vi "Dashboard Main.vi"() -> ()   [LabVIEW 2019]
uses:
  Program Files (x86)/National Instruments/LabVIEW 2019/examples/Design Patterns/Queued Message Handler/support/QMH Fundamentals - Message Cluster.ctl
  <vilib>/Utility/miscctls.llb/LVRowAndColumnTypeDef.ctl
  <vilib>/event_ctls.llb/eventvkey.ctl
  src robot/TypeDefs/Falcon Temperatures.ctl
  <vilib>/Rock Robotics/WPI/Dashboard/WPI_DashboardLogging Global.vi
  <vilib>/Rock Robotics/Network Tables/NT Read Numeric Array.vi
  <vilib>/Rock Robotics/Network Tables/NT Read Boolean.vi
  <vilib>/Rock Robotics/Network Tables/NT Write Boolean.vi
  Personalities Tool/Personalities Tool.lvlib
  91361502-ee7e-4c80-8d6f-41942abc4405.vi
panel:
  in  "Mini View Toolbar":bool
  in  "Mini View Button":bool
  out "Boolean 5":bool
  in  "Boolean 4":bool
  in  "Developer Settings":bool
  in  "Match Ready":bool
  in  "Left Sidebar Expanded":bool
  in  "Left Sidebar Mini":bool
  in  "Minimized Toolbar Button":bool
  out "Tab Control 2":enum32{"Page 1", "Page 2"}(tab)
  out "Numeric 3":dbl
  out "String 5":string
  out "New Throttle 2":bool
  out "Highest Temp Label 3":string
  out "Highest Temp Label 4":string
  in  "Flywheel Velocity - 2":bool
  in  "Flywheel Velocity Plus 2":bool
  out "String 7":string
  out "String 8":string
  out "String 6":string
  out "Numeric 2":dbl
  out "String":string
  out "Widger Manager":enum32{"Page 1", "Page 2"}(tab)
  out "String 2":string
  out "String 3":string
  in  "Flywheel Velocity Plus":bool
  in  "Flywheel Velocity -":bool
  out "Highest Temp Label":string
  out "String 4":string
  out "Highest Temp Label 2":string
  out "New Throttle":bool
  in  "Boolean":bool
  out "Tab Control":enum32{"Page 1", "Page 3", "Page 2"}(tab)
  in  "Exanded View Toolbar":bool
  in  "stop 2":bool
  out "# elements in queue 2":i32
  out "Elapsed Time (s)":dbl
  out "# elements in queue":i32
  in  "TCP":refnum<k5>
  in  "Rec Mode":enum32{"Stop", "Record", "Playback"}(radio)
  out "Robot IP":string
  out "Image Message":string="Timeout in Camera Communications"
  in  "Dashboard Tab":T1(tab)
  out "Right follow":dbl
  out "Left follow":dbl
  out "Turret":dbl
  out "Right Lead":dbl
  out "Left lead":dbl
  out "Flywheel":dbl
  out "Flywheel Velocity":dbl
  in  "Select Auto":string(combo)="Select Autonomous ..."
  out "NT Connection":bool
  out "Mode":T2(ring)=enum."Auto Disabled"
  out "Accelerator":dbl format="%#_6f"
  in  "Shooter Trim +":bool
  in  "DB/String 9":string
  in  "DB/String 8":string
  in  "DB/String 7":string
  in  "DB/String 6":string
  in  "DB/String 5":string
  in  "DB/String 4":string
  in  "DB/String 3":string
  in  "DB/String 2":string
  in  "DB/String 1":string
  in  "DB/String 0":string
  in  "DB/Slider 0":dbl(slide) scale=0.0..5.0
  in  "DB/Slider 1":dbl(slide) scale=0.0..5.0
  in  "DB/Slider 2":dbl(slide) scale=0.0..5.0
  in  "DB/Slider 3":dbl(slide) scale=0.0..5.0
  out "DB/LED 3":bool
  out "DB/LED 2":bool
  out "DB/LED 1":bool
  out "DB/LED 0":bool
  in  "DB/Button 3":bool
  in  "DB/Button 2":bool
  in  "DB/Button 1":bool
  in  "DB/Button 0":bool caption="New Name"
  in  "Launch Personalities Tool":bool
  in  "Test Slider":dbl(slide) scale=0.0..100.0 scale format="%#_3g"
  in  "On/Off":bool caption="Solenoid"
  in  "Test Name":u16(ring) items=["Select the test to run..."]
  in  "Test Tree":string(tree)
  in  "Motor":cluster{"Value":dbl, "Enable":bool} {"Value" scale=-1.0..1.0 scale format="%#_3g"}
  out "Progress":T3 {"Test Progress" scale=0.0..100.0}
  in  "Rev/Fwd":cluster{"Forward":bool, "Reverse":bool}
  in  "Test Ring":u16(ring) items=["Monochrome", "Color"]
  out "Cmd Status":string
  in  "Execute Command":bool
  in  "Command Params":string[][](table)
  in  "Command Selection":i32(listbox)
  in  "CheckList":i32(listbox)
  out "Tree":string(tree)
  # "o"
  # "F"
  # "o"
  # "F"
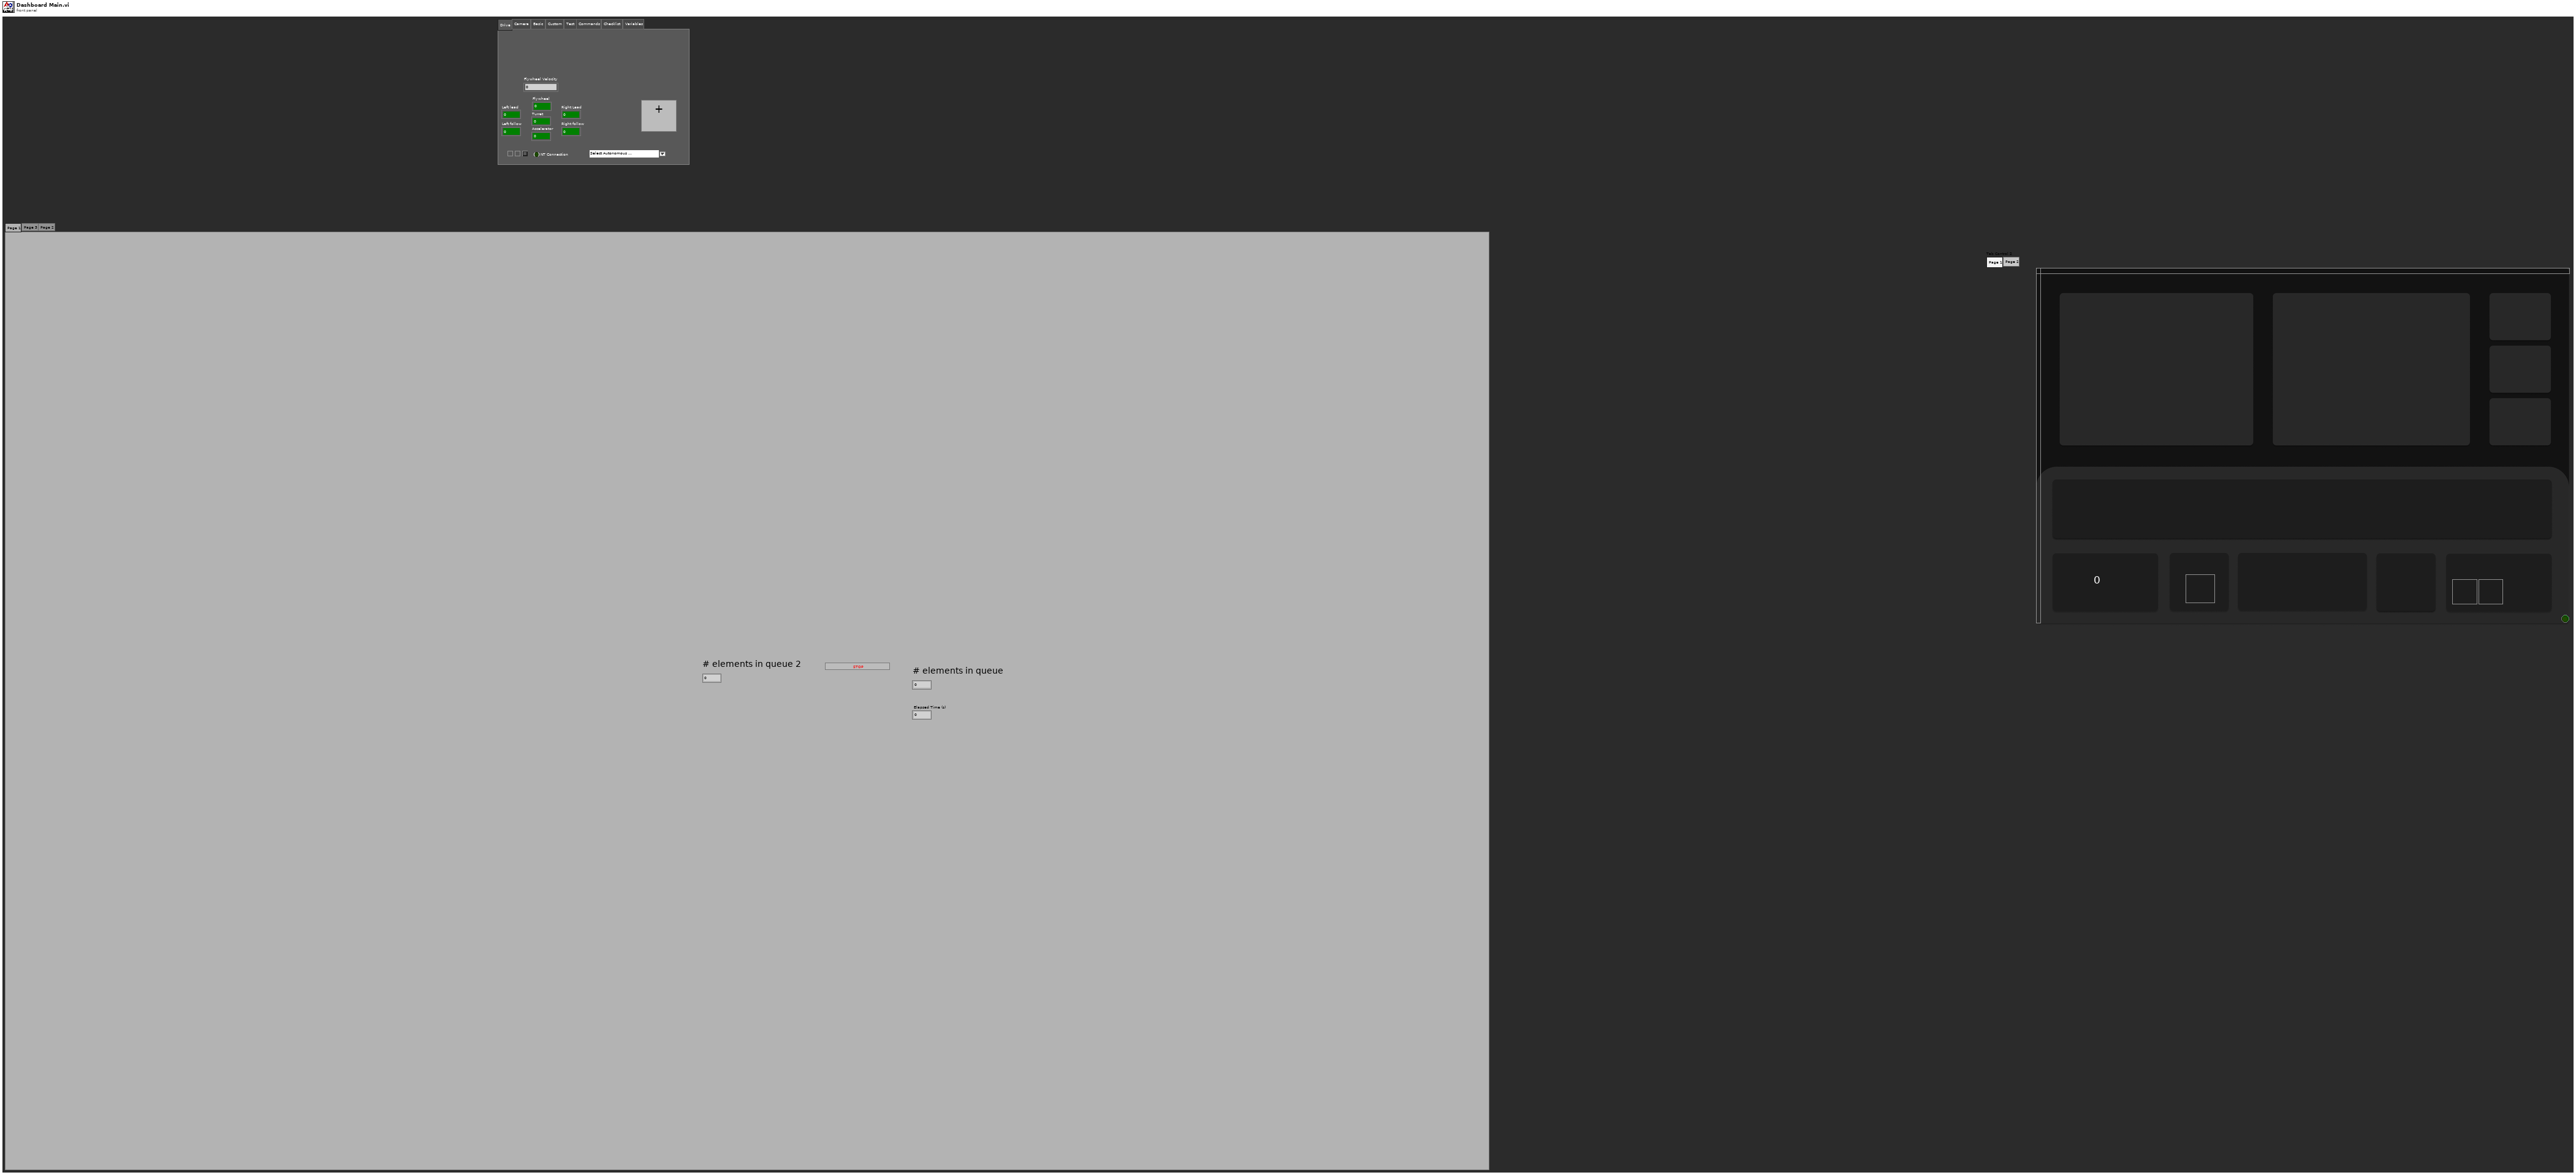
[diagram p1: front panel]
types:
  T1 = enum32{"Drive", "Camera", "Basic", "Custom", "Test", "Commands", "Checklist", "Variables"}
  T2 = enum8{"Tele-Op Disabled", "Tele-Op Enabled", "Auto Disabled", "Auto Enabled", "Test Disabled", "Test Enabled", "Disconnected", "No Code", "E-Stop"}
  T3 = cluster{"Test Progress":u8, "Test Progress Text":string}
  T4 = typedef "QMH Fundamentals - Message Cluster.ctl" = cluster{"Message":string, "Message Data":variant}
  T5 = cluster{"IDs":cluster{"RPC field ID":u16, "Unique ID":u16}, "String":string}
  T6 = typedef "Falcon Temperatures.ctl" = enum16{"Accelerator", "Turret", "Flywheel", "Right follow", "Right lead", "Left follow", "Left lead"}
  T7 = cluster{"Error Strings":string, "Disable Counts":cluster{u16, u16}, "Rail Faults":cluster{u16, u16, u16}, "Robot IP":string, "DB Mode":u8, "Event Info":cluster{"Name":string, "Type":u8, "Number":u16, "Replay":u8}}
  T8 = cluster{"Storage":cluster{"Disk Free":u64, "RAM Block":u32, "RAM free":u32}, "CPU Utilization":cluster{"CPU % ISR":sgl, "CPU % Time Crit":sgl, "CPU % Timed Str":sgl, "CPU % High":sgl, "CPU % Above":sgl, "CPU % Normal":sgl, "CPU % Low":sgl}, "CAN":cluster{"% Bus Utilization":sgl, "Bus Off Cnt":u32, "TX_FIFO Full Cnt":u32, "Receive Error Cnt":u8, "Transmit Error Cnt":u8}, "HID":cluster{"HID Outputs":u32, "Rumble Low":u16, "Rumble High":u16}[]}
  T9 = cluster{"Status bits":cluster{"Test Mode":bool, "Autonomous":bool, "Enabled":bool, "Code Start":bool, "Brownout":bool, "Reserved 2":bool, "Reserved 3":bool, "E-Stop":bool}, "Code Trace":cluster{"Disabled":bool, "TeleOp":bool, "Auto":bool, "Test":bool}, "Controller Type":enum16{"unknown", "cRIO", "roboRio"}, "Code?":enum16{"unknown", "noCode", "code"}, "Battery V":dbl}
  T10 = cluster{"Operation":enum16{"Update", "Clear"}, "Color Box":u32}[]
  T11 = typedef "eventvkey.ctl" = enum16{"ASCII", "Enter", "Return", "Shift", "Ctrl", "Alt", "Cmd", "Opt", "Caps", "NumLock", "Clear", "Break", "Up", "Down", "Left", "Right", "Insert", "Delete", "Home", "End", "PageUp", "PageDown", "Escape", "Help", "Pause", "ScrollLock", "F1", "F2", "F3", "F4", "F5", "F6", "F7", "F8", "F9", "F10", "F11", "F12", "F13", "F14", "F15", "F16", "F17", "F18", "F19", "F20", "F21", "F22", "F23", "F24", "Play", "VolumeUp", "VolumeDown", "Mute", "Two Byte Char"}
  T12 = cluster{"Image Size":bool, "Image Type":bool, "Pixel Value":bool, "ROI Information":bool, "Zoom Factor":bool}
  T13 = cluster{"Operation":enum16{"Update", "Clear"}, "Color Box":u32}
  T14 = typedef "LVRowAndColumnTypeDef.ctl" = cluster{"Row":i32, "Column":i32}
  T15 = cluster{"Shift":bool, "Ctrl":bool, "Alt":bool, "Cmd":bool, "Opt":bool}
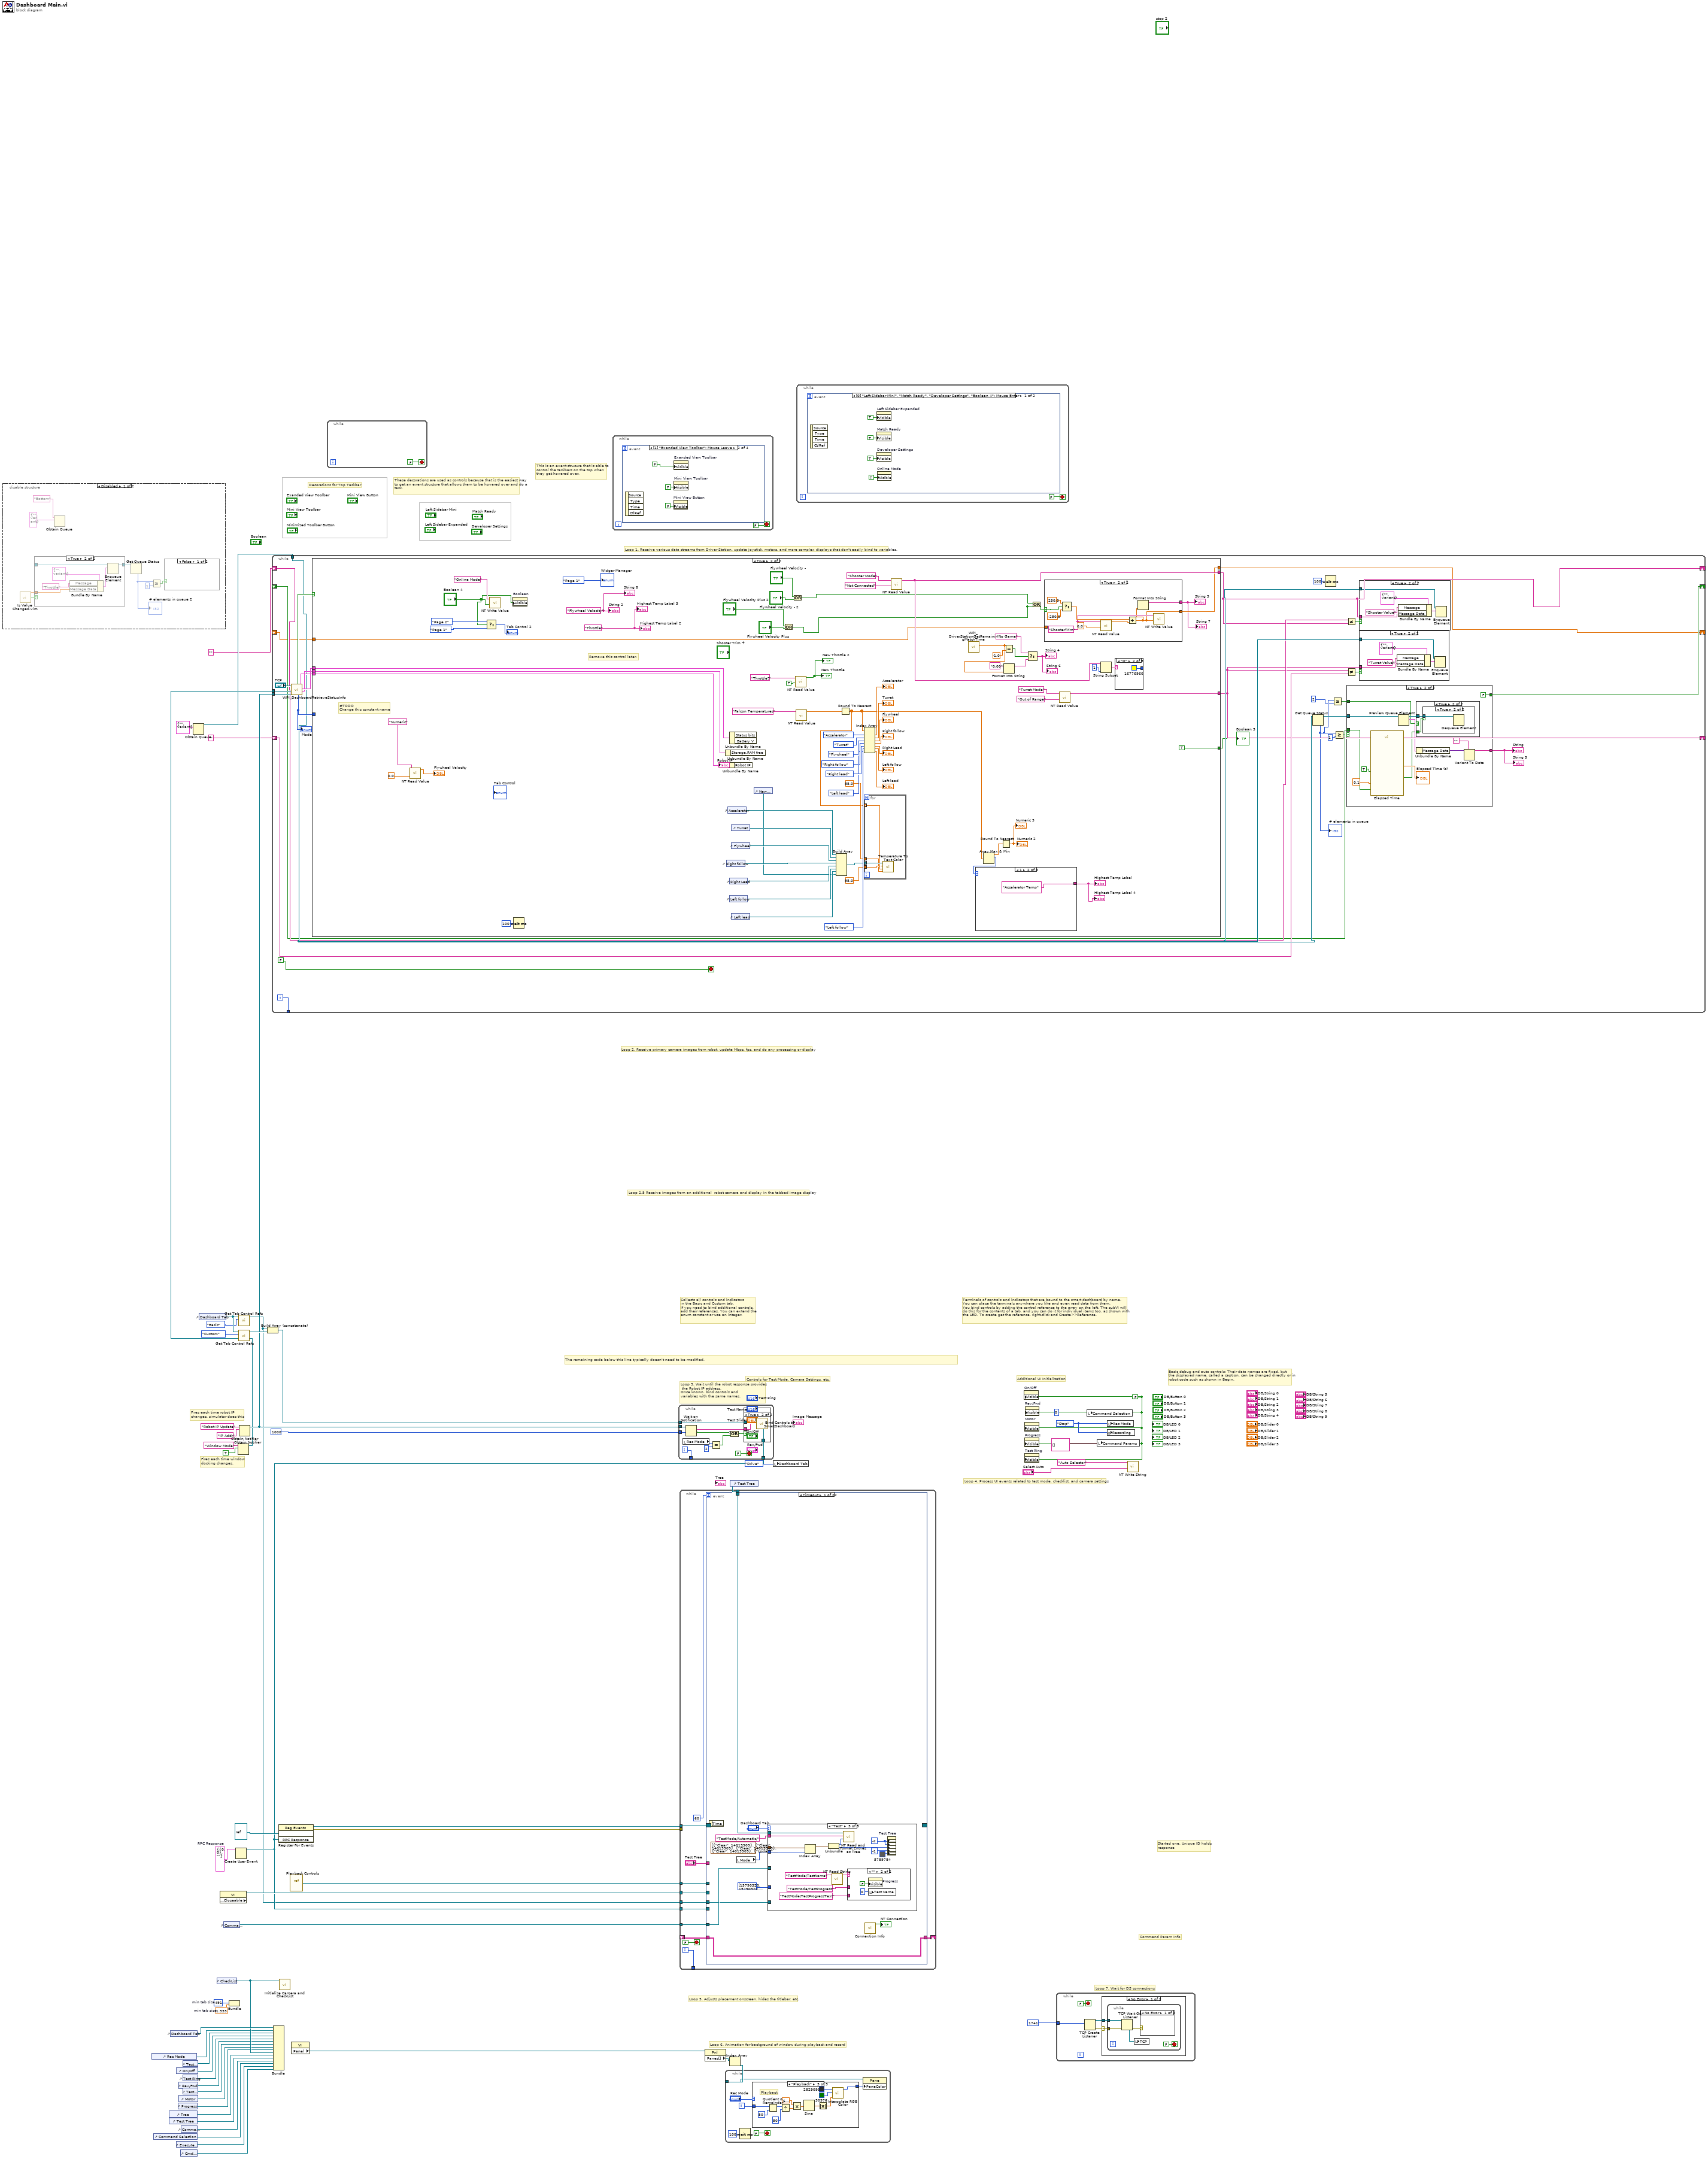
[diagram p0: block diagram]
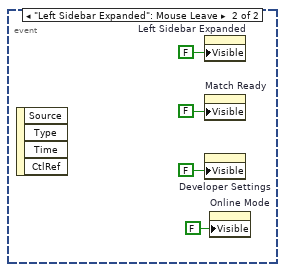
[diagram p2: hidden frame]
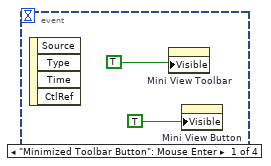
[diagram p3: hidden frame]
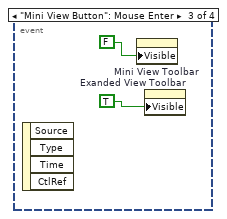
[diagram p4: hidden frame]
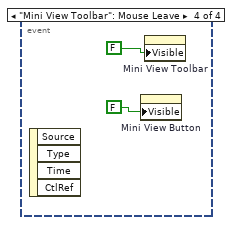
[diagram p5: hidden frame]
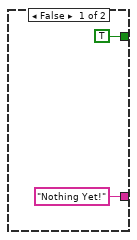
[diagram p9: hidden frame]
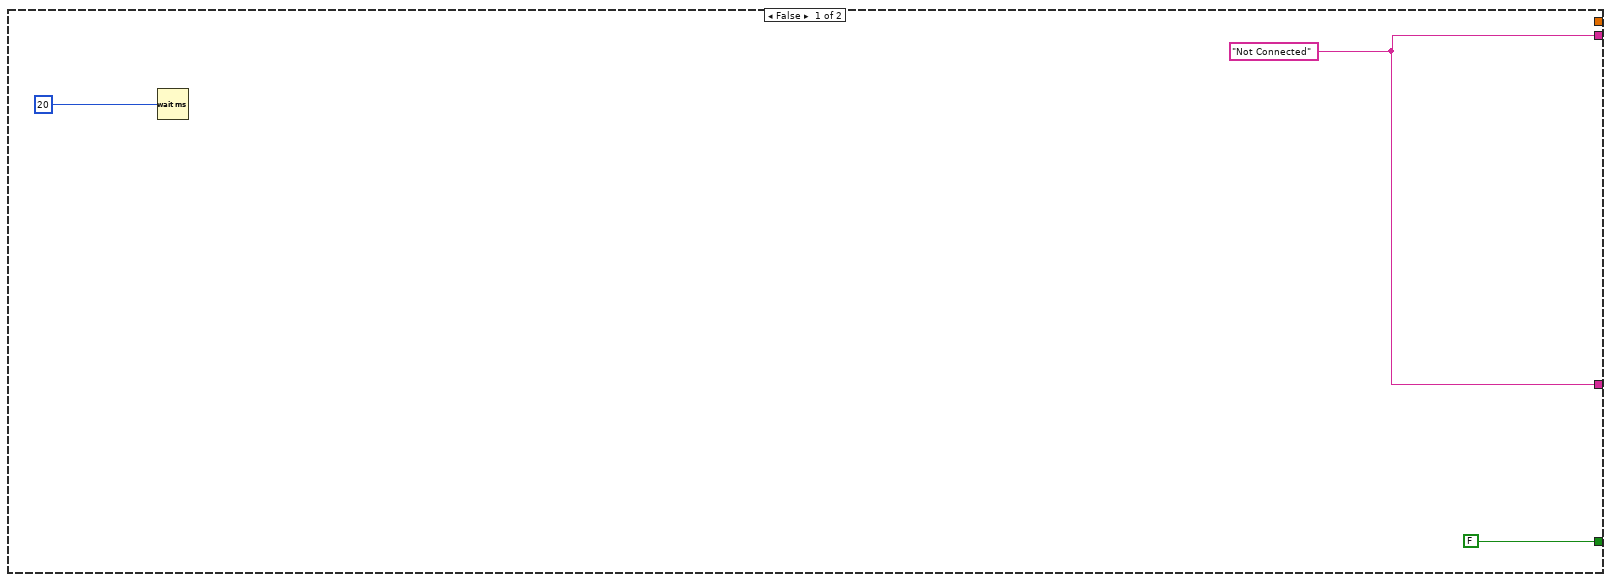
[diagram p14: hidden frame]
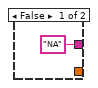
[diagram p15: hidden frame]
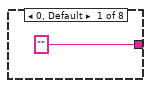
[diagram p16: hidden frame]
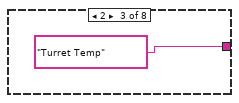
[diagram p17: hidden frame]
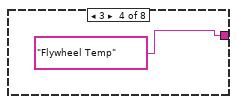
[diagram p18: hidden frame]
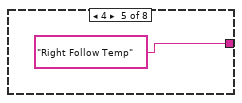
[diagram p19: hidden frame]
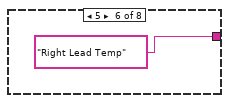
[diagram p20: hidden frame]
diagram:
  w16 = T5 {"IDs"={"RPC field ID"=0, "Unique ID"=0}, "String"=""}  # RPC Response
  w36 = 491  # min tab size
  w35 = 1.333  # min tab size
  w42 = enum32{"Stop", "Record", "Playback"}."Stop" ("Rec Mode")
  w23 = FALSE ("Visible")
  # "This is an event strucure that is able to\ncontrol the taskbars on the top when \nthey get hovered over."
  # "Decorations for Top Taskbar"
  # "These decorations are used as controls because that is the easiest way to get an event structure that allows them to be hovered over and do a task."
  # "Loop 2.5 Receive images from an additional  robot camera and display in the tabbed image display"
  # "Command Param Info"
  # "Started one, Unique ID holds\nresponse"
  # "Loop 7. Wait for DS connections"
  # "Basic debug and auto controls: Their data names are fixed, but\nthe displayed name, called a caption, can be changed directly or in\nrobot code such as shown in Begin."
  # "Controls for Test Mode, Camera Settings, etc."
  # "Additional UI Initialization"
  # "Loop 6. Animation for background of window during playback and record"
  # "Fires each time robot IP\nchanges, simulator does this"
  # "Fires each time window\ndocking changes."
  # "Collects all controls and indicators\nin the Basic and Custom tab.\nIf you need to bind additional controls,\nadd their references. You can extend the\nenum constant or use an integer."
  # "The remaining code below this line typically doesn't need to be modified."
  # "Loop 4. Process UI events related to test mode, checklist, and camera settings"
  # "Terminals of controls and indicators that are bound to the smart dashboard by name.\nYou can place the terminals anywhere you like and even read data from them.\nYou bind controls by adding the control reference to the array on the left. The subVI will\ndo this for the contents of a tab, and you can do it for individual items too, as shown with\nthe LED. To create get the reference, right-click and Create>>Reference."
  # "Loop 3. Wait until the robot response provides\n the Robot IP address.\nOnce known, bind controls and\nvariables with the same names."
  # "Loop 5. Adjusts placement onscreen, hides the titlebar, etc."
  # "Loop 1. Receive various data streams from Driver Station, update joystick, motors, and more complex displays that don't easily bind to variables."
  # "Loop 2. Receive primary camera images from robot, update Mbps, fps, and do any processing or display"
  n1 = disable-structure shown="Disabled" {
    frame Disabled {
      n2 = Obtain Queue(name (unnamed)="Bottom", element data type=T4 {"Message"="", "Message Data"=variant} ("Message Cluster")) -> ()  [unwired: 3 in, 3 out]
      n3 = call "Is Value Changed.vim"("value"=w61) -> ("changed or first call?"=w59:bool)
      n4 = case shown="True" w59 {
        tunnel: [_ w67] -> w61
        tunnel: _ -> [w64 w66]
        tunnel: [w64 w65] -> w58
        frame False {
        }
        frame True {
          n5 = Bundle By Name(cluster=T4 {"Message"="", "Message Data"=variant} ("element"), "Message"="Throttle", "Message Data"=w67) -> (w70:T4)
          n6 = Enqueue Element(queue=w66, element=w70) -> (queue out=w65:refnum<queue>)  [unwired: 2 in, 2 out]
        }
      }
      n7 = Get Queue Status(queue=w58) -> (# elements in queue=w57:i32)  [unwired: 2 in, 7 out]
      "# elements in queue 2" <- w57
      n8 = Greater Or Equal?(x=w57, y=1) -> (x >= y?=w60:bool)
      n9 = case shown="False" w60 {
        frame False {
        }
        frame True {
        }
      }
    }
    frame Enabled {
    }
  }
  n10 = control-ref of="Rec Mode"() -> (w29:refnum<vi>)
  n11 = control-ref of="Command Selection"() -> (w15:refnum<vi>)
  n12 = control-ref of="Tree"() -> (w33:refnum<vi>)
  n13 = control-ref of="Test Tree"() -> (w32:refnum<vi>)
  n14 = control-ref of="Dashboard Tab"() -> (w37:refnum<vi>)
  n15 = control-ref of="Execute Command"() -> (w17:refnum<vi>)
  n16 = control-ref of="On/Off"() -> (w27:refnum<vi>)
  n17 = control-ref of="Progress"() -> (w24:refnum<vi>)
  n18 = control-ref of="Rev/Fwd"() -> (w25:refnum<vi>)
  n19 = control-ref of="Motor"() -> (w30:refnum<vi>)
  n20 = control-ref of="Cmd Status"() -> (w11:refnum<vi>)
  n21 = control-ref of="Command Params"() -> (w18:refnum<vi>)
  n22 = control-ref of="Test Slider"() -> (w28:refnum<vi>)
  n23 = control-ref of="Test Ring"() -> (w26:refnum<vi>)
  n24 = control-ref of="Test Name"() -> (w31:refnum<vi>)
  n25 = Obtain Queue(element data type=T4 {"Message"="", "Message Data"=variant} ("Message Cluster")) -> (queue out=w3:refnum<queue>)  [unwired: 4 in, 2 out]
  n26 = control-ref of="Dashboard Tab"() -> (w40:refnum<vi>)
  n27 = control-ref of="CheckList"() -> (w34:refnum<vi>)
  n28 = property class="VI" props=["Front Panel.Closeable"]() -> (reference out=w41:refnum<vi>)  [unwired: 2 in, 2 out]
  n29 = control-ref of="Command Params"() -> (w10:refnum<vi>)
  n30 = Bundle("min tab size"=w36, "min tab size"=w35) -> ()  [unwired: 1 in, 1 out]
  n31 = Create User Event(user event datatype=w16) -> (user event=w12:refnum<user-event>)  [unwired: 1 in, 1 out]
  n32 = Obtain Notifier(name (unnamed)="Window Mode", notification data type=TRUE) -> (notifier out=w21:refnum<notifier>)  [unwired: 2 in, 2 out]
  n33 = call <vilib>:"Get Tab Control Refs.vi"("Page Index"=T1."Basic" ("Dashboard Tab"), "TabControl in"=w40) -> ("ControlsOnPage"=w9:refnum<vi>[])  [unwired: 9 in]
  n34 = call <vilib>:"Get Tab Control Refs.vi"("Page Index"=T1."Custom" ("Dashboard Tab"), "TabControl in"=w40) -> ("ControlsOnPage"=w39:refnum<vi>[])  [unwired: 9 in]
  n35 = Obtain Notifier(name (unnamed)="Robot IP Update", notification data type="IP Addr" ("name (unnamed)")) -> (notifier out=w22:refnum<notifier>)  [unwired: 2 in, 2 out]
  n36 = Build Array (concatenate)(w9, w39) -> (w38:refnum<vi>[])
  n37 = while {
    tunnel: [w99] -> _
    tunnel: w22 -> [w94]
    tunnel: w21 -> [w91]
    tunnel: w3 -> [w90]
    shift-right: [w79] -> _
    shift-left: "" -> [w89]
    shift-right: [w80] -> _
    shift-left: "" -> [w88]
    shift-right: [w78] -> _
    shift-left: _ -> [w87]
    shift-right: [w73] -> _
    shift-left: _ -> [w72]
    i -> [w99]
    stop <- FALSE stop-if-true
    n38 = call <vilib>:"WPI_DashboardRetrieveStatusInfo.vi"("Binding Refnum"=w94, "Window Mode Notifier"=w91, "TCP Cnx"="TCP") -> ("Power and Errors"=w95:T7, "Robot Metrics"=w97:T8, "Status Info"=w98:T9, "Robot Mode"=w93:T2, "Process?"=w96:bool)  [unwired: 3 in, 1 out]
    "Mode" <- w93
    n39 = case shown="True" w96 {
      tunnel: w98 -> [_ w207]
      tunnel: w97 -> [_ w206]
      tunnel: w95 -> [_ w205]
      tunnel: w93 -> [_ _]
      tunnel: [FALSE ("Boolean") TRUE ("Boolean")] -> w77
      tunnel: [w129 w160] -> w79
      tunnel: [w129 w159] -> w80
      tunnel: [_ w151] -> w73
      tunnel: w72 -> [_ w150]
      frame False {
        w129 = "Not Connected" ("String")
        n40 = Wait (ms)(milliseconds to wait=u32 20) -> ()  [unwired: 1 out]
      }
      frame True {
        w133 = "Throttle" ("Highest Temp Label 2")
        w132 = "Flywheel Velocity" ("String 2")
        # "Remove this control later."
        # "#TODO\nChange this constant name"
        n41 = call-poly <vilib>:"NT Read Value.vi"("Default Value"=0.0, "Name"="Numeric") -> ("Numeric"=→"Flywheel Velocity":dbl)  [unwired: 8 in, 1 out]
        n42 = Select(t=enum32{"Page 1", "Page 2"}."Page 2" ("Tab Control 2"), s="Boolean 4", f=enum32{"Page 1", "Page 2"}."Page 1" ("Tab Control 2")) -> (s? t:f=→"Tab Control 2":enum32{"Page 1", "Page 2"})
        n43 = call-poly <vilib>:"NT Write Value.vi"("Boolean"="Boolean 4", "Name"="Online Mode") -> ()  [unwired: 9 in, 1 out]
        n44 = property on="Boolean" class="Bool (strict)"("Visible"="Boolean 4") -> ()  [unwired: 2 in, 2 out]
        n45 = Wait (ms)(milliseconds to wait=u32 100) -> ()  [unwired: 1 out]
        n46 = Unbundle By Name(w206) -> ()  [unwired: 1 out]
        n47 = control-ref of="Right follow"() -> (w175:refnum<vi>)
        n48 = control-ref of="Accelerator"() -> (w181:refnum<vi>)
        n49 = Unbundle By Name(w205) -> ("Robot IP"=→"Robot IP":string)
        n50 = control-ref of="Right Lead"() -> (w174:refnum<vi>)
        n51 = control-ref of="Left follow"() -> (w173:refnum<vi>)
        n52 = Unbundle By Name(w207) -> ()  [unwired: 2 out]
        n53 = control-ref of="Turret"() -> (w180:refnum<vi>)
        n54 = control-ref of="Flywheel"() -> (w176:refnum<vi>)
        n55 = control-ref of="Left lead"() -> (w172:refnum<vi>)
        n56 = control-ref of="New Dashboard Temp Indicator"() -> (w158:refnum<vi>)
        n57 = Or(x="Flywheel Velocity Plus 2", y="Flywheel Velocity Plus") -> (x .or. y?=w139:bool)
        n58 = Or(x="Flywheel Velocity -", y="Flywheel Velocity - 2") -> (x .or. y?=w141:bool)
        n59 = call-poly <vilib>:"NT Read Value.vi"("Default Value"=FALSE, "Name"="Throttle?") -> ("Boolean"=→"New Throttle" →"New Throttle 2":bool)  [unwired: 8 in, 1 out]
        n60 = call-poly <vilib>:"NT Read Value.vi"("Name"="Falcon Temperatures") -> ("Numeric Array"=w194:dbl[])  [unwired: 9 in, 1 out]
        n61 = Build Array(w181, w180, w176, w175, w174, w173, w172, w158) -> (w179:refnum<vi>[])
        n62 = Round To Nearest(number=w194) -> (nearest integer value=w163:dbl[])
        n63 = Index Array(array=w163, index #1=Falcon_Temperatures."Accelerator" ("Enum"), index #2=Falcon_Temperatures."Turret" ("Enum"), index #3=Falcon_Temperatures."Flywheel" ("Enum"), index #4=Falcon_Temperatures."Right follow" ("Enum"), index #5=Falcon_Temperatures."Right lead" ("Enum"), index #6=Falcon_Temperatures."Left follow" ("Enum"), index #7=Falcon_Temperatures."Left lead" ("Enum")) -> (element #1=→"Accelerator":dbl, element #2=→"Turret":dbl, element #3=→"Flywheel":dbl, element #4=→"Right follow":dbl, element #5=→"Right Lead":dbl, element #6=→"Left follow":dbl, element #7=→"Left lead":dbl)
        n64 = for {
          tunnel: w179 -> [w229] mode=indexing
          tunnel: w163 -> [w228] mode=indexing
          tunnel: 95.0 ("Upper Limit") -> [w227]
          tunnel: 85.0 ("Lower Limit") -> [w226]
          n65 = call "Temperature To Text Color.vi"("Lower Limit"=w226, "Temperature"=w228, "Upper Limit"=w227, "reference"=w229) -> ()  [unwired: 8 in]
        }
        n66 = call-poly <vilib>:"NT Read Value.vi"("Default Value"="Not Connected", "Name"="Shooter Mode") -> ("String"=w159:string)  [unwired: 8 in, 1 out]
        n67 = call <vilib>:"WPI_DriverStationGetRemainingMatchTime.vi"() -> ("Match Time(s)"=w154:sgl)  [unwired: 10 in, 1 out]
        n68 = Array Max & Min(array=w163) -> (max value=w167:dbl, max index (indices)=w166:i32)  [unwired: 2 out]
        n69 = case shown="1" w166 {
          tunnel: ["" "Accelerator Temp" "Turret Temp" "Flywheel Temp" "Right Follow Temp" "Right Lead Temp" "Left Follow Temp" "Left Lead Temp"] -> w134
          frame 0, Default {
          }
          frame 1 {
          }
          frame 2 {
          }
          frame 3 {
          }
          frame 4 {
          }
          frame 5 {
          }
          frame 6 {
          }
          frame 7 {
          }
        }
        "Highest Temp Label" <- w134
        "Highest Temp Label 4" <- w134
        n70 = Round To Nearest(number=w167) -> (nearest integer value=→"Numeric 2" →"Numeric 3":dbl)
        n71 = Format Into String(initial string="0:00", w154) -> (resulting string=w153:string)  [unwired: 2 in, 1 out]
        n72 = Equal?(x=w154, y=sgl -1.0) -> (x = y?=w156:bool)
        n73 = Select(t="No Game", s=w156, f=w153) -> (s? t:f=→"String 4" →"String 6":string)
        n74 = Or(x=w141, y=w139) -> ()  [unwired: 1 out]
        n75 = case shown="True" w139 {
          selector: w139 -> [_ w211]
          tunnel: ["NA" w210] -> w135
          tunnel: [_ w209] -> w151
          tunnel: w150 -> [_ _]
          frame False {
          }
          frame True {
            w212 = "ShooterTrim" ("Name")
            n76 = Select(t=250.0, s=w211, f=-250.0) -> (s? t:f=w215:dbl)
            n77 = call-poly <vilib>:"NT Read Value.vi"("Default Value"=0.0, "Name"=w212) -> ("Numeric"=w214:dbl)  [unwired: 8 in, 1 out]
            n78 = Add(x=w215, y=w214) -> (x+y=w209:dbl)
            n79 = Format Into String(w209) -> (resulting string=w210:string)  [unwired: 3 in, 1 out]
            n80 = call-poly <vilib>:"NT Write Value.vi"("Numeric"=w209, "Name"=w212) -> ()  [unwired: 9 in, 1 out]
          }
        }
        "String 3" <- w135
        "String 7" <- w135
        n81 = call-poly <vilib>:"NT Read Value.vi"("Default Value"="Out of Range", "Name"="Turret Mode") -> ("String"=w160:string)  [unwired: 8 in, 1 out]
        n82 = String Subset(string=w159, length (rest)=1 ("length (rest)")) -> (substring=w203:string)  [unwired: 1 in]
        n83 = case shown="\"D\"" w203 {
          tunnel: [u32 16711680 ("Text.Text Colors:BG Color") u32 16776960 ("Text.Text Colors:BG Color") u32 65280 ("Text.Text Colors:BG Color")] -> _
          frame "N", Default {
          }
          frame "D" {
          }
          frame "B", "F", "M" {
          }
        }
        "Highest Temp Label 2" <- w133
        "String 2" <- w132
        "Widger Manager" <- enum32{"Page 1", "Page 2"}."Page 1" ("Widger Manager")
        "Highest Temp Label 3" <- w133
        "String 8" <- w132
      }
    }
    "Boolean 5" <- w77
    n84 = Get Queue Status(queue=w90) -> (queue out=w81:refnum<queue>, # elements in queue=w76:i32)  [unwired: 2 in, 6 out]
    "# elements in queue" <- w76
    n85 = Wait (ms)(milliseconds to wait=u32 100) -> ()  [unwired: 1 out]
    n86 = Greater Or Equal?(x=w76, y=2) -> (x >= y?=w74:bool)
    n87 = Greater Or Equal?(x=w76, y=1) -> (x >= y?=w82:bool)
    n88 = Not Equal?(x=w88, y=w80) -> (x != y?=w85:bool)
    n89 = Not Equal?(x=w79, y=w89) -> (x != y?=w84:bool)
    n90 = case shown="True" w82 {
      tunnel: ["Nothing Yet!" w114] -> w71
      tunnel: w81 -> [_ w112]
      tunnel: [TRUE FALSE ("Auto Reset")] -> w78
      tunnel: w87 -> [_ w106]
      tunnel: w74 -> [_ w104]
      frame False {
      }
      frame True {
        n91 = call "Elapsed Time"("Time Target (s)"=0.1, "Reset"=w106, "Auto Reset"=TRUE) -> ("Elapsed Time (s)"=→"Elapsed Time (s)":dbl, "Time has Elapsed"=w103:bool)  [unwired: 9 in, 6 out]
        n92 = Preview Queue Element(queue=w112) -> (queue out=w110:refnum<queue>, element=w111:T4)  [unwired: 2 in, 2 out]
        n93 = case shown="True" w104 {
          tunnel: w110 -> [_ w117]
          tunnel: w103 -> [_ w116]
          frame False {
          }
          frame True {
            n94 = case shown="True" w116 {
              tunnel: w117 -> [_ w118]
              frame False {
              }
              frame True {
                n95 = Dequeue Element(queue=w118) -> ()  [unwired: 2 in, 4 out]
              }
            }
          }
        }
        n96 = Unbundle By Name(w111) -> ("Message Data"=w113:variant)
        n97 = Variant To Data(type="", Variant=w113) -> (data=w114:string)  [unwired: 1 in, 1 out]
      }
    }
    "String" <- w71
    "String 5" <- w71
    n98 = case shown="True" w85 {
      tunnel: w90 -> [_ w125]
      tunnel: w80 -> [_ w124]
      frame False {
      }
      frame True {
        n99 = Bundle By Name(cluster=T4 {"Message"="", "Message Data"=variant} ("element"), "Message"="Shooter Value", "Message Data"=w124) -> (w128:T4)
        n100 = Enqueue Element(queue=w125, element=w128) -> ()  [unwired: 2 in, 3 out]
      }
    }
    n101 = case shown="True" w84 {
      tunnel: w79 -> [_ w120]
      tunnel: w90 -> [_ w119]
      frame False {
      }
      frame True {
        n102 = Bundle By Name(cluster=T4 {"Message"="", "Message Data"=variant} ("element"), "Message"="Turret Value", "Message Data"=w120) -> (w123:T4)
        n103 = Enqueue Element(queue=w119, element=w123) -> ()  [unwired: 2 in, 3 out]
      }
    }
  }
  n104 = Bundle("Dashboard Tab"=w37, "Rec Mode"=w29, "Test Slider"=w28, "On/Off"=w27, "Test Ring"=w26, "Rev/Fwd"=w25, "Test Name"=w31, "Motor"=w30, "Progress"=w24, "CheckList"=w34, "Tree"=w33, "Test Tree"=w32, "Command Params"=w18, "Command Selection"=w15, "Execute Command"=w17, "Cmd Status"=w11) -> ()  [unwired: 1 in, 1 out]
  n105 = register-events(refnum<vi> refnum, w12) -> (reference out=w46:refnum<event-registration>, error out=w45:errorcluster)  [unwired: 2 in]
  n106 = call "Initialize Camera and CheckList.vi"("ListBox in"=w34) -> ()  [unwired: 11 in]
  n107 = vi-ref "Playback Controls.vi"() -> (w47:refnum<vi>)
  n108 = property class="VI"() -> ("Panel"=w49:refnum<vi>)  [unwired: 2 in, 2 out]
  n109 = while {
    stop <- FALSE stop-if-true
  }
  n110 = while {
    stop <- FALSE stop-if-true
    n111 = event shown="[1] \"Exanded View Toolbar\": Mouse Leave" {
      selector: _ -> [_ _ _ _]
      dyn-events: _ -> [_ _ _ _]
      timeout: _ -> [_ _ _ _]
      event "Minimized Toolbar Button": Mouse Enter {
        n112 = event-data() -> ()  [unwired: 1 in, 4 out]
        n113 = property on="Mini View Toolbar" class="Bool (strict)"("Visible"=TRUE) -> ()  [unwired: 2 in, 2 out]
        n114 = property on="Mini View Button" class="Bool (strict)"("Visible"=TRUE) -> ()  [unwired: 2 in, 2 out]
      }
      event "Exanded View Toolbar": Mouse Leave {
        n115 = event-data() -> ()  [unwired: 1 in, 4 out]
        n116 = property on="Mini View Button" class="Bool (strict)"("Visible"=FALSE) -> ()  [unwired: 2 in, 2 out]
        n117 = property on="Exanded View Toolbar" class="Bool (strict)"("Visible"=FALSE) -> ()  [unwired: 2 in, 2 out]
        n118 = property on="Mini View Toolbar" class="Bool (strict)"("Visible"=FALSE) -> ()  [unwired: 2 in, 2 out]
      }
      event "Mini View Button": Mouse Enter {
        n119 = event-data() -> ()  [unwired: 1 in, 4 out]
        n120 = property on="Mini View Toolbar" class="Bool (strict)"("Visible"=FALSE) -> ()  [unwired: 2 in, 2 out]
        n121 = property on="Exanded View Toolbar" class="Bool (strict)"("Visible"=TRUE) -> ()  [unwired: 2 in, 2 out]
      }
      event "Mini View Toolbar": Mouse Leave {
        n122 = event-data() -> ()  [unwired: 1 in, 4 out]
        n123 = property on="Mini View Button" class="Bool (strict)"("Visible"=FALSE) -> ()  [unwired: 2 in, 2 out]
        n124 = property on="Mini View Toolbar" class="Bool (strict)"("Visible"=FALSE) -> ()  [unwired: 2 in, 2 out]
      }
    }
  }
  n125 = while {
    tunnel: w38 -> [w255]
    tunnel: w22 -> [w253]
    tunnel: [w251] -> _
    tunnel: u32 1000 ("milliseconds to wait") -> [w250]
    tunnel: w12 -> [w244]
    i -> [w251]
    stop <- FALSE stop-if-true
    n126 = local read "Rec Mode"() -> (w246:enum32{"Stop", "Record", "Playback"})
    n127 = Wait on Notification(notifier=w253, timeout in ms (-1)=w250) -> (notification=w252:string, timed out?=w248:bool)  [unwired: 2 in, 2 out]
    n128 = Equal?(x=w246, y=u16 2 ("Rec Mode")) -> (x = y?=w247:bool)
    n129 = Compound Arithmetic op=OR(invert w248, w247) -> (w249:bool)
    n130 = case shown="True" w249 {
      tunnel: w255 -> [_ w258]
      tunnel: w252 -> [_ w257]
      tunnel: w244 -> [_ w256]
      frame False {
      }
      frame True {
        n131 = call <vilib>:"Bind Controls to SmartDashboard.vi"("RPC ref"=w256, "Bound Control Refs"=w258, "Server IP Address"=w257) -> ()  [unwired: 9 in]
      }
    }
  }
  n132 = property class="Pnl"(reference=w49) -> ("Panes[]"=w50:refnum<vi>[])  [unwired: 1 in, 2 out]
  n133 = Index Array(array=w50) -> (element=w48:refnum<vi>)  [unwired: 1 in]
  n134 = while {
    tunnel: w48 -> [w260]
    i -> [w263]
    stop <- FALSE stop-if-true
    n135 = Wait (ms)(milliseconds to wait=u32 100) -> ()  [unwired: 1 out]
    n136 = case shown="\"Playback\"" "Rec Mode" {
      tunnel: w263 -> [_ _ w278]
      tunnel: [u32 2829099 ("Base Color") u32 11141120 ("Target Color") w267] -> w259
      frame "Stop", Default {
        # "Reset the color, extra updates don't cost much"
      }
      frame "Record" {
      }
      frame "Playback" {
        # "Playback"
        n137 = Quotient & Remainder(x=w278, y=u32 50 ("milliseconds to wait")) -> (x-y*floor(x/y)=w274:u32)  [unwired: 1 out]
        n138 = Divide(x=w274, y=u32 50 ("milliseconds to wait")) -> (x/y=w271:dbl)
        n139 = Multiply(x=6.283185307179586, y=w271) -> (x*y=w276:dbl)
        n140 = Sine(x=w276) -> (sin(x)=w275:dbl)
        n141 = Absolute Value(x=w275) -> (abs(x)=w268:dbl)
        n142 = call "Interpolate RGB Color.vi"("Proportion"=w268, "Target Color"=u32 30976, "Base Color"=u32 2829099) -> ("Result Color"=w267:u32)  [unwired: 8 in]
      }
    }
    n143 = property class="Pane"(reference=w260, "PaneColor"=w259) -> ()  [unwired: 1 in, 2 out]
  }
  n144 = control-ref of="Test Tree"() -> (w51:refnum<vi>)
  n145 = while {
    tunnel: [w288] -> _
    tunnel: w51 -> [w287]
    tunnel: w47 -> [w286]
    tunnel: w46 -> [w285]
    tunnel: w45 -> [_]
    tunnel: w41 -> [w284]
    tunnel: w12 -> [w283]
    tunnel: w10 -> [w282]
    shift-right: [w281] -> _
    shift-left: _ -> [w280]
    tunnel: w9 -> [w279]
    i -> [w288]
    stop <- FALSE stop-if-true
    n146 = event shown="[0] Timeout" {
      selector: w285 -> [_ _ _ _ _ _ _ _ _ _ _ _ _ _ _ _ _ _ _ _ _ _]
      dyn-events: [_ _ _ _ _ _ _ _ _ _ _ _ _ _ _ _ _ w549 _ _ _ _] -> _
      timeout: u32 60 ("milliseconds to wait") -> [_ _ _ _ _ _ _ _ _ _ _ _ _ _ _ _ _ _ _ _ _ _]
      tunnel: w287 -> [w300 _ _ _ _ _ _ _ _ _ _ _ _ _ _ _ _ _ _ _ _ _]
      tunnel: "Test Tree" -> [_ _ _ _ _ _ _ _ _ _ _ _ w518 w526 w528 w532 w540 _ _ _ _ _]
      tunnel: w286 -> [_ _ _ _ _ _ _ _ _ _ _ _ _ _ _ _ _ w551 _ w569 _ _]
      tunnel: w284 -> [_ _ _ _ _ _ _ _ _ _ _ _ _ _ _ _ _ w547 _ _ _ _]
      tunnel: w283 -> [_ _ _ _ _ _ _ _ _ _ _ _ _ _ _ _ _ w545 _ _ _ _]
      tunnel: w282 -> [w295 _ _ _ _ _ _ w469 _ _ _ _ _ _ _ _ _ _ _ _ _ _]
      tunnel: [w294 w344 w346 w448 w453 w462 w466 w467 w476 w486 w493 w505 w517 w524 w527 w531 w539 w544 w564 w566 w570 w583] -> w281
      tunnel: w280 -> [w294 w344 w346 w448 w453 w462 w466 w467 _ _ w493 w505 w517 w524 w527 w531 w539 w544 w564 w566 w570 w583]
      tunnel: w279 -> [w292 _ _ _ _ _ _ _ _ _ _ _ _ _ _ _ _ _ _ _ _ _]
      event Timeout {
        n147 = event-data() -> ()  [unwired: 1 in, 1 out]
        n148 = local read "Mode"() -> (w297:T2)
        n149 = case shown="\"Test\"" "Dashboard Tab" {
          tunnel: w300 -> [_ _ w316 _ _]
          tunnel: "TestMode/Automatic/" ("Name Pattern") -> [_ _ w315 _ _]
          tunnel: T10 [{"Operation"=enum."Clear", "Color Box"=14013909}, {"Operation"=enum."Clear", "Color Box"=14013909}, {"Operation"=enum."Clear", "Color Box"=14013909}, {"Operation"=enum."Clear", "Color Box"=14013909}, {"Operation"=enum."Update", "Color Box"=14013909}, {"Operation"=enum."Update", "Color Box"=16777215}, {"Operation"=enum."Clear", "Color Box"=14013909}, {"Operation"=enum."Clear", "Color Box"=14013909}, {"Operation"=enum."Clear", "Color Box"=14013909}] -> [_ _ w308 _ w336]
          tunnel: w297 -> [_ _ w307 _ w335]
          tunnel: u32[] [15790320, 15790320, 15790320, 15790320, 16777215, 16777215, 15790320, 15790320, 15790320] -> [_ _ _ _ w341]
          tunnel: w295 -> [_ _ _ _ w329]
          tunnel: w292 -> [_ w302 _ _ _]
          frame "Custom", Default {
          }
          frame "Basic" {
            n150 = call <vilib>:"WPI_DashboardUpdateNames.vi"("Controls on Tab"=w302) -> ()  [unwired: 11 in]
          }
          frame "Test" {
            w314 = -2 ("Active Item:Row Number")
            n151 = Index Array(array=w308, index=w307) -> (element=w309:T13)
            n152 = Unbundle(w309) -> ("Operation"=w310:enum16{"Update", "Clear"}, "Color Box"=w311:u32)
            n153 = call <vilib>:"NT Read String.vi"("Name"="TestMode/TestName") -> ("String"=w305:string)  [unwired: 9 in, 1 out]
            n154 = call <vilib>:"NT Read and Format Entries as Tree.vi"("Operation"=w310, "Name Pattern"=w315, "Tree Refnum"=w316) -> ()  [unwired: 7 in, 2 out]
            n155 = case shown="\"\"" w305 {
              tunnel: "TestMode/TestProgress" ("Name") -> [w318 _]
              tunnel: "TestMode/TestProgressText" ("Name") -> [w317 _]
              frame Default {
                n156 = call <vilib>:"NT Read Number.vi"("Name"=w318) -> ("Numeric"=w319:dbl)  [unwired: 9 in, 1 out]
                n157 = call <vilib>:"NT Read String.vi"("Name"=w317) -> ("String"=w320:string)  [unwired: 9 in, 1 out]
                n158 = Bundle("Numeric"=w319, "String"=w320) -> (→"Progress":cluster{"Numeric":dbl, "String":string})  [unwired: 1 in]
              }
              frame "" {
                n159 = property on="Progress" class="Clust (strict)"("Visible"=FALSE) -> ()  [unwired: 2 in, 2 out]
                n160 = local write "Test Name"(u16 0) -> ()
              }
            }
            n161 = property on="Test Tree" class="Tree (strict)"("Active Item Row Number"=w314, "ActiveColNum"=w314, "CellBG"=w311, "Active Item Row Number"=-1 ("Active Item:Row Number"), "CellBG"=u32 5789784 ("Color Box")) -> ()  [unwired: 2 in, 2 out]
          }
          frame "Variables" {
            w326 = string[] ["CameraPublisher", "Usage", "DB"]  # Items to initially close
            n162 = First Call?() -> (First Call?: T/F=w327:bool)
            n163 = control-ref of="Tree"() -> (w328:refnum<vi>)
            n164 = Select(t=w326, s=w327, f=string[] []) -> (s? t:f=w324:string[])
            n165 = call <vilib>:"NT Read and Format Entries as Tree.vi"("Tags to  Close"=w324, "Tree Refnum"=w328) -> ()  [unwired: 8 in, 2 out]
          }
          frame "Commands" {
            w337 = u32 5789784 ("Color Box")
            w338 = T14 {"Row"=-1, "Column"=-2} ("Active Cell:Active Cell")
            w340 = T14 {"Row"=-2, "Column"=-2} ("Active Cell:Active Cell")
            n166 = Index Array(array=w341, index=w335) -> (element=w339:u32)
            n167 = Index Array(array=w336, index=w335) -> (element=w334:T13)
            n168 = Unbundle(w334) -> ("Operation"=w333:enum16{"Update", "Clear"})  [unwired: 1 out]
            n169 = local read "Command Selection"() -> (w332:i32)
            n170 = property on="Command Selection" class="MCListbox (strict)"("ActiveCell"=w340, "CellBG"=w339, "ActiveCell"=w338, "CellBG"=w337) -> ()  [unwired: 2 in, 2 out]
            n171 = call <vilib>:"WPI_DashboardUpdate RPC Info.vi"("Operation"=w333) -> ("update"=w331:bool, "commands"=w330:string[][])  [unwired: 9 in]
            n172 = property on="Command Selection" class="MCListbox (strict)"("ItemNames"=w330) -> ()  [unwired: 2 in, 2 out]
            n173 = property on="Command Params" class="Tbl (strict)"("Active Cell"=w340, "Cell BG Color"=w339, "Active Cell"=w338, "Cell BG Color"=w337) -> ()  [unwired: 2 in, 2 out]
            n174 = call <vilib>:"WPI_DashboardUpdate Command Params.vi"("Update"=w331, "NewVal"=w332, "Commands"=w330, "Param Tbl"=w329) -> ()  [unwired: 7 in, 1 out]
          }
        }
        n175 = call <vilib>:"Connextion Info.vi"() -> ("Connected"=→"NT Connection":bool)  [unwired: 10 in, 1 out]
      }
      event "Launch Personalities Tool": Value Change {
        n176 = event-data() -> ()  [unwired: 1 in, 6 out]
        n177 = call "Launch Personalities Tool.vi"() -> ("error out"=w343:errorcluster)  [unwired: 11 in]
        n178 = call <vilib>:"General Error Handler.vi"("error in (no error)"=w343) -> ()  [unwired: 10 in, 5 out]
        n179 = local write "Launch Personalities Tool"(FALSE ("Launch Personalities Tool")) -> ()
      }
      event "Test Tree": Value Change {
        # "Show appropriate\ncontrols"
        n180 = event-data() -> ("CtlRef"=w349:refnum<vi>, "NewVal"=w347:string)  [unwired: 1 in]
        n181 = call <vilib>:"WPI_UtilitiesGetTreeIOName.vi"("NewVal"=w347, "TreeControl in"=w349) -> ("I/O Name"=w350:string)  [unwired: 9 in]
        n182 = case shown="\"Camera\"" w350 {
          selector: w350 -> [_ w357 _ w379 w388 _]
          tunnel: w347 -> [_ _ w376 w378 _ w395]
          tunnel: cluster{string[]}[] [{["640x480", "320x240", "160x120"]}, {["Auto", "Fixed indoor", "Fixed outdoor 1", "Fixed outdoor 2", "Fixed fluorescent 1", "Fixed fluorescent 2", "Hold current"]}, {["Auto", "Flicker-free 50 Hz", "Flicker-free 60 Hz", "Hold current"]}, {["None", "Prioritize frame rate", "Prioritize image quality"]}, {["Monochrome", "Color"]}] -> [_ _ _ _ _ w394]
          frame Default {
            w352 = FALSE ("Visible")
            w351 = FALSE ("Visible")
            n183 = property on="Motor" class="Clust (strict)"("Visible"=w351) -> ()  [unwired: 2 in, 2 out]
            n184 = property on="Test Ring" class="Ring (strict)"("Visible"=w351) -> ()  [unwired: 2 in, 2 out]
            n185 = property on="Rev/Fwd" class="Clust (strict)"("Visible"=w352) -> ()  [unwired: 2 in, 2 out]
            n186 = property on="On/Off" class="Bool (strict)"("Visible"=w352) -> ()  [unwired: 2 in, 2 out]
            n187 = property on="Test Slider" class="Slide (strict)"("Visible"=w352) -> ()  [unwired: 2 in, 2 out]
          }
          frame "Analog Out", "Motor", "PWM" {
            w358 = FALSE ("Visible")
            n188 = case shown="\"Analog Out\"" w357 {
              tunnel: [1.0 ("Value") -1.0 ("Value") 0.0 ("Value")] -> w356
              tunnel: [255.0 ("Value") 1.0 ("Value") 5.0 ("Value")] -> w355
              tunnel: [128.0 ("Value") 0.0 ("Value") 0.0 ("Value")] -> w354
              tunnel: [64.0 ("Value") 0.5 ("Value") 1.0 ("Value")] -> w353
              frame "PWM" {
              }
              frame "Motor", Default {
              }
              frame "Analog Out" {
              }
            }
            n189 = property on="Motor" class="Clust (strict)"("Visible"=TRUE) -> ()  [unwired: 2 in, 2 out]
            n190 = property on="Value" class="Slide (strict)"("Value"=w354, "Scale.Minimum"=w356, "Scale.Maximum"=w355, "Scale.Increment"=w353) -> ()  [unwired: 2 in, 2 out]
            n191 = property on="On/Off" class="Bool (strict)"("Visible"=w358) -> ()  [unwired: 2 in, 2 out]
            n192 = property on="Test Slider" class="Slide (strict)"("Visible"=w358) -> ()  [unwired: 2 in, 2 out]
            n193 = property on="Test Ring" class="Ring (strict)"("Visible"=w358) -> ()  [unwired: 2 in, 2 out]
            n194 = property on="Rev/Fwd" class="Clust (strict)"("Visible"=w358) -> ()  [unwired: 2 in, 2 out]
          }
          frame "Servo" {
            w374 = FALSE ("Visible")
            n195 = call <vilib>:"NT Read Number.vi"("Name"=w376) -> ("Numeric"=w375:dbl)  [unwired: 9 in, 1 out]
            n196 = property on="Test Slider" class="Slide (strict)"("Visible"=TRUE, "Scale.Maximum"=170.0 ("Scale.Range:Maximum")) -> ()  [unwired: 2 in, 2 out]
            n197 = local write "Test Slider"(w375) -> ()
            n198 = property on="Motor" class="Clust (strict)"("Visible"=w374) -> ()  [unwired: 2 in, 2 out]
            n199 = property on="Rev/Fwd" class="Clust (strict)"("Visible"=w374) -> ()  [unwired: 2 in, 2 out]
            n200 = property on="On/Off" class="Bool (strict)"("Visible"=w374) -> ()  [unwired: 2 in, 2 out]
            n201 = property on="Test Ring" class="Ring (strict)"("Visible"=w374) -> ()  [unwired: 2 in, 2 out]
          }
          frame "Relay", "Solenoid" {
            w377 = FALSE ("Visible")
            n202 = property on="Motor" class="Clust (strict)"("Visible"=w377) -> ()  [unwired: 2 in, 2 out]
            n203 = property on="Test Slider" class="Slide (strict)"("Visible"=w377) -> ()  [unwired: 2 in, 2 out]
            n204 = Search and Replace String(input string=w378, search string="/Value  **", replace string="/Direction") -> (result string=w384:string)  [unwired: 5 in, 3 out]
            n205 = property on="Test Ring" class="Ring (strict)"("Visible"=w377) -> ()  [unwired: 2 in, 2 out]
            n206 = call <vilib>:"NT Read String.vi"("Name"=w384) -> ("String"=w382:string)  [unwired: 9 in, 1 out]
            n207 = Equal?(x="Both directions", y=w382) -> (x = y?=w380:bool)
            n208 = Not(x=w380) -> (.not. x?=w381:bool)
            n209 = property on="Rev/Fwd" class="Clust (strict)"("Visible"=w380) -> ()  [unwired: 2 in, 2 out]
            n210 = property on="On/Off" class="Bool (strict)"("Visible"=w381, "Caption.Text"=w379) -> ()  [unwired: 2 in, 2 out]
          }
          frame "Compressor", "Digital Out" {
            w387 = FALSE ("Visible")
            # "Get direction and finish"
            n211 = property on="Motor" class="Clust (strict)"("Visible"=w387) -> ()  [unwired: 2 in, 2 out]
            n212 = property on="Test Slider" class="Slide (strict)"("Visible"=w387) -> ()  [unwired: 2 in, 2 out]
            n213 = property on="Test Ring" class="Ring (strict)"("Visible"=w387) -> ()  [unwired: 2 in, 2 out]
            n214 = property on="On/Off" class="Bool (strict)"("Visible"=TRUE, "Caption.Text"=w388) -> ()  [unwired: 2 in, 2 out]
            n215 = property on="Rev/Fwd" class="Clust (strict)"("Visible"=FALSE) -> ()  [unwired: 2 in, 2 out]
          }
          frame "Camera" {
            n216 = call <vilib>:"Get Last Path Segment.vi"("String in"=w395) -> ("String out"=w396:string)  [unwired: 10 in]
            n217 = property on="On/Off" class="Bool (strict)"("Visible"=FALSE) -> ()  [unwired: 2 in, 2 out]
            n218 = property on="Motor" class="Clust (strict)"("Visible"=FALSE) -> ()  [unwired: 2 in, 2 out]
            n219 = property on="Rev/Fwd" class="Clust (strict)"("Visible"=FALSE) -> ()  [unwired: 2 in, 2 out]
            n220 = case shown="\"White Balance  **\"" w396 {
              tunnel: w395 -> [w402 w411 w420 w429 w438 _ w444]
              tunnel: w394 -> [w400 w408 w417 w426 w435 _ _]
              frame "Size  **" {
                n221 = Index Array(array=w400) -> (element=w399:cluster{string[]})  [unwired: 1 in]
                n222 = call <vilib>:"NT Read String.vi"("Name"=w402) -> ("String"=w401:string)  [unwired: 9 in, 1 out]
                n223 = Unbundle(w399) -> (w397:string[])
                n224 = Match First String(2:w397, 3:w401) -> (0:w398:i32)  [unwired: 1 out]
                n225 = property on="Test Ring" class="Ring (strict)"("Value"=w398, "Strings []"=w397) -> ()  [unwired: 2 in, 2 out]
                n226 = property on="Test Ring" class="Ring (strict)"("Visible"=TRUE) -> ()  [unwired: 2 in, 2 out]
                n227 = property on="Test Slider" class="Slide (strict)"("Visible"=FALSE) -> ()  [unwired: 2 in, 2 out]
              }
              frame "White Balance  **" {
                n228 = Index Array(array=w408, index=1) -> (element=w409:cluster{string[]})
                n229 = call <vilib>:"NT Read String.vi"("Name"=w411) -> ("String"=w410:string)  [unwired: 9 in, 1 out]
                n230 = Unbundle(w409) -> (w406:string[])
                n231 = Match First String(2:w406, 3:w410) -> (0:w405:i32)  [unwired: 1 out]
                n232 = property on="Test Ring" class="Ring (strict)"("Value"=w405, "Strings []"=w406) -> ()  [unwired: 2 in, 2 out]
                n233 = property on="Test Ring" class="Ring (strict)"("Visible"=TRUE) -> ()  [unwired: 2 in, 2 out]
                n234 = property on="Test Slider" class="Slide (strict)"("Visible"=FALSE) -> ()  [unwired: 2 in, 2 out]
              }
              frame "Exposure  **" {
                n235 = Index Array(array=w417, index=2) -> (element=w418:cluster{string[]})
                n236 = call <vilib>:"NT Read String.vi"("Name"=w420) -> ("String"=w419:string)  [unwired: 9 in, 1 out]
                n237 = Unbundle(w418) -> (w414:string[])
                n238 = Match First String(2:w414, 3:w419) -> (0:w415:i32)  [unwired: 1 out]
                n239 = property on="Test Ring" class="Ring (strict)"("Value"=w415, "Strings []"=w414) -> ()  [unwired: 2 in, 2 out]
                n240 = property on="Test Ring" class="Ring (strict)"("Visible"=TRUE) -> ()  [unwired: 2 in, 2 out]
                n241 = property on="Test Slider" class="Slide (strict)"("Visible"=FALSE) -> ()  [unwired: 2 in, 2 out]
              }
              frame "Exposure Priority  **" {
                n242 = Index Array(array=w426, index=3) -> (element=w427:cluster{string[]})
                n243 = call <vilib>:"NT Read String.vi"("Name"=w429) -> ("String"=w428:string)  [unwired: 9 in, 1 out]
                n244 = Unbundle(w427) -> (w423:string[])
                n245 = Match First String(2:w423, 3:w428) -> (0:w424:i32)  [unwired: 1 out]
                n246 = property on="Test Ring" class="Ring (strict)"("Value"=w424, "Strings []"=w423) -> ()  [unwired: 2 in, 2 out]
                n247 = property on="Test Ring" class="Ring (strict)"("Visible"=TRUE) -> ()  [unwired: 2 in, 2 out]
                n248 = property on="Test Slider" class="Slide (strict)"("Visible"=FALSE) -> ()  [unwired: 2 in, 2 out]
              }
              frame "Color Enable  **" {
                n249 = Index Array(array=w435, index=4) -> (element=w436:cluster{string[]})
                n250 = call <vilib>:"NT Read String.vi"("Name"=w438) -> ("String"=w437:string)  [unwired: 9 in, 1 out]
                n251 = Unbundle(w436) -> (w432:string[])
                n252 = Match First String(2:w432, 3:w437) -> (0:w433:i32)  [unwired: 1 out]
                n253 = property on="Test Ring" class="Ring (strict)"("Value"=w433, "Strings []"=w432) -> ()  [unwired: 2 in, 2 out]
                n254 = property on="Test Ring" class="Ring (strict)"("Visible"=TRUE) -> ()  [unwired: 2 in, 2 out]
                n255 = property on="Test Slider" class="Slide (strict)"("Visible"=FALSE) -> ()  [unwired: 2 in, 2 out]
              }
              frame Default {
                n256 = property on="Test Ring" class="Ring (strict)"("Visible"=FALSE) -> ()  [unwired: 2 in, 2 out]
                n257 = property on="Test Slider" class="Slide (strict)"("Visible"=FALSE) -> ()  [unwired: 2 in, 2 out]
              }
              frame "Brightness  **", "Color Level  **", "Compression  **", "FPS  **", "Sharpness  **" {
                n258 = call <vilib>:"NT Read Number.vi"("Name"=w444) -> ("Numeric"=w443:dbl)  [unwired: 9 in, 1 out]
                n259 = local write "Test Slider"(w443) -> ()
                n260 = property on="Test Slider" class="Slide (strict)"("Visible"=TRUE, "Scale.Maximum"=100.0 ("Scale.Range:Maximum")) -> ()  [unwired: 2 in, 2 out]
                n261 = property on="Test Ring" class="Ring (strict)"("Visible"=FALSE) -> ()  [unwired: 2 in, 2 out]
              }
            }
          }
        }
        n262 = property on="Progress" class="Clust (strict)"("Visible"=FALSE) -> ()  [unwired: 2 in, 2 out]
      }
      event "Test Name": Mouse Enter {
        # "Populate the ring with the list of tests"
        n263 = event-data() -> ()  [unwired: 1 in, 1 out]
        n264 = call <vilib>:"NT Read String Array.vi"("Name"="TestMode/TestList") -> ("String Array"=w452:string[])  [unwired: 9 in, 1 out]
        n265 = Build Array (concatenate)("Select the test to run...", w452) -> (w451:string[])
        n266 = property on="Test Name" class="Ring (strict)"("Strings []"=w451) -> ()  [unwired: 2 in, 2 out]
      }
      event "Test Name": Value Change {
        w454 = FALSE ("Visible")
        # "Tell the robot the test name to run"
        n267 = event-data() -> ("NewVal"=w458:u16)  [unwired: 1 in]
        n268 = property on="Test Name" class="Ring (strict)"() -> ("Strings []"=w459:string[])  [unwired: 2 in, 2 out]
        n269 = local write "Progress"(T3 {"Test Progress"=0, "Test Progress Text"=""} ("Progress")) -> ()
        n270 = Index Array(array=w459, index=w458) -> (element=w457:string)
        n271 = call <vilib>:"NT Write String.vi"("String"=w457, "Name"="TestMode/TestName") -> ()  [unwired: 9 in, 1 out]
        n272 = property on="Progress" class="Clust (strict)"("Visible"=TRUE) -> ()  [unwired: 2 in, 2 out]
        n273 = property on="Motor" class="Clust (strict)"("Visible"=w454) -> ()  [unwired: 2 in, 2 out]
        n274 = property on="Test Slider" class="Slide (strict)"("Visible"=w454) -> ()  [unwired: 2 in, 2 out]
        n275 = property on="On/Off" class="Bool (strict)"("Visible"=w454) -> ()  [unwired: 2 in, 2 out]
        n276 = property on="Rev/Fwd" class="Clust (strict)"("Visible"=w454) -> ()  [unwired: 2 in, 2 out]
        n277 = property on="Test Ring" class="Ring (strict)"("Visible"=w454) -> ()  [unwired: 2 in, 2 out]
      }
      event "Select Auto": Mouse Enter {
        # "Populate the combo box with the list of autonomous options"
        n278 = event-data() -> ()  [unwired: 1 in, 1 out]
        n279 = call <vilib>:"NT Read String Array.vi"("Name"="Auto List") -> ("String Array"=w461:string[])  [unwired: 9 in, 1 out]
        n280 = property on="Select Auto" class="CmbBox"("Strings[]"=w461) -> ()  [unwired: 2 in, 2 out]
      }
      event "Select Auto": Value Change {
        # "User modified the Auto Selection. Write to NT variable so robot knows."
        n281 = event-data() -> ("NewVal"=w464:string)  [unwired: 1 in]
        n282 = call <vilib>:"NT Write String.vi"("String"=w464, "Name"="Auto Selector") -> ()  [unwired: 9 in, 1 out]
      }
      event "Command Selection": Value Change {
        # "Get the params and show in table"
        n283 = event-data() -> ("NewVal"=w470:i32)  [unwired: 1 in]
        n284 = property on="Command Selection" class="MCListbox (strict)"() -> ("ItemNames"=w468:string[][])  [unwired: 2 in, 2 out]
        n285 = call <vilib>:"WPI_DashboardUpdate Command Params.vi"("NewVal"=w470, "Commands"=w468, "Param Tbl"=w469) -> ()  [unwired: 8 in, 1 out]
      }
      event "Execute Command": Value Change {
        # "Started one, Unique ID holds\nresponse"
        n286 = event-data() -> ()  [unwired: 1 in, 1 out]
        n287 = property on="Command Selection" class="MCListbox (strict)"() -> ("ItemNames"=w481:string[][])  [unwired: 2 in, 2 out]
        n288 = Index Array(array=w481, index (row)="Command Selection", index (col)=0) -> (element=w479:string)
        n289 = call <vilib>:"Invoke Commands.vi"("Command Params"="Command Params", "Function Name"=w479) -> ("Params"=w475:u8, "Started"=w474:bool)  [unwired: 7 in, 1 out]
        n290 = Array Subset(array="Command Params", length (row)=w475) -> (w476:string[][])  [unwired: 3 in]
        n291 = Select(t="Executing" ("Cmd Status"), s=w474, f="" ("Cmd Status")) -> (s? t:f=→"Cmd Status":string)
      }
      event "Command Selection": Double Click {
        n292 = event-data() -> ("Row"=w489:i32)  [unwired: 1 in]
        n293 = property on="Command Selection" class="MCListbox (strict)"() -> ("ItemNames"=w492:string[][])  [unwired: 2 in, 2 out]
        n294 = local read "Command Params"() -> (w488:string[][])
        n295 = Index Array(array=w492, index (row)=w489, index (col)=0) -> (element=w490:string)
        n296 = call <vilib>:"Invoke Commands.vi"("Command Params"=w488, "Function Name"=w490) -> ("Params"=w487:u8, "Started"=w482:bool)  [unwired: 7 in, 1 out]
        n297 = Array Subset(array=w488, length (row)=w487) -> (w486:string[][])  [unwired: 3 in]
        n298 = Select(t="Executing" ("Cmd Status"), s=w482, f="" ("Cmd Status")) -> (s? t:f=w483:string)
        n299 = local write "Cmd Status"(w483) -> ()
      }
      event "CheckList": Double Click {
        # "Shift clears all"
        # "Update symbols on the listbox"
        n300 = event-data() -> ("PlatMods.Shift"=w494:bool, "Row"=w496:i32)  [unwired: 1 in]
        n301 = case shown="True" w494 {
          tunnel: w496 -> [w500 _]
          tunnel: 1 -> [w499 _]
          frame False {
            n302 = property on="CheckList" class="LstBox (strict)"() -> ("Item Symbols"=w498:i32[])  [unwired: 2 in, 2 out]
            n303 = Replace Array Subset(array=w498, new element=w499, index=w500) -> (w497:i32[])
            n304 = property on="CheckList" class="LstBox (strict)"("Item Symbols"=w497) -> ()  [unwired: 2 in, 2 out]
          }
          frame True {
            w501 = 0 ("Top Row")
            n305 = property on="CheckList" class="LstBox (strict)"() -> ("Number of Rows"=w503:u32)  [unwired: 2 in, 2 out]
            n306 = Initialize Array(0, w503) -> (w502:i32[])
            n307 = property on="CheckList" class="LstBox (strict)"("Top Row"=w501, "Value"=w501, "Item Symbols"=w502) -> ()  [unwired: 2 in, 2 out]
          }
        }
      }
      event "CheckList": Key Down {
        # "Update symbols on the listbox\nLeft and right keys check and uncheck"
        n308 = event-data() -> ("VKey"=w507:T11)  [unwired: 1 in]
        n309 = case shown="\"Left\", \"Right\"" w507 {
          selector: w507 -> [w512 _]
          tunnel: eventvkey."Left" ("VKey") -> [w510 _]
          frame "Left", "Right" {
            n310 = Equal?(x=w510, y=w512) -> (x = y?=w511:bool)
            n311 = Select(t=0, s=w511, f=1) -> (s? t:f=w513:i32)
            n312 = property on="CheckList" class="LstBox (strict)"() -> ("Item Symbols"=w516:i32[])  [unwired: 2 in, 2 out]
            n313 = Replace Array Subset(array=w516, new element=w513, index="CheckList") -> (w515:i32[])
            n314 = property on="CheckList" class="LstBox (strict)"("Item Symbols"=w515) -> ()  [unwired: 2 in, 2 out]
          }
          frame Default {
          }
        }
      }
      event "Motor.Enable": Value Change {
        # "When the test mode otor enable helper is set, update that\ntree row item's value"
        n315 = event-data() -> ("NewVal"=w522:bool)  [unwired: 1 in]
        n316 = Unbundle("Motor") -> ("Value"=w521:dbl)  [unwired: 1 out]
        n317 = Select(t=w521, s=w522, f=0.0) -> (s? t:f=w519:dbl)
        n318 = call <vilib>:"NT Write Number.vi"("Numeric"=w519, "Name"=w518) -> ()  [unwired: 9 in, 1 out]
      }
      event "Test Slider": Value Change {
        # "When the test mode slider helper is set, update that\ntree row item's value"
        n319 = event-data() -> ("NewVal"=w525:dbl)  [unwired: 1 in]
        n320 = call <vilib>:"NT Write Number.vi"("Numeric"=w525, "Name"=w526) -> ()  [unwired: 9 in, 1 out]
      }
      event "On/Off": Value Change {
        # "When the test mode on/off helper value is set, update that\ntree row item's value"
        n321 = event-data() -> ("NewVal"=w530:bool)  [unwired: 1 in]
        n322 = Boolean To (0,1)(Boolean=w530) -> (0, 1=w529:i16)
        n323 = call <vilib>:"NT Write Number.vi"("Numeric"=w529, "Name"=w528) -> ()  [unwired: 9 in, 1 out]
      }
      event "Rev/Fwd": Value Change {
        # "When the test mode helper value for relays is set, update that\ntree row item's value"
        n324 = event-data() -> ("NewVal.Forward"=w538:bool, "NewVal.Reverse"=w537:bool)  [unwired: 1 in]
        n325 = Boolean To (0,1)(Boolean=w538) -> (0, 1=w534:i16)
        n326 = Boolean To (0,1)(Boolean=w537) -> (0, 1=w536:i16)
        n327 = Negate(x=w536) -> (-x=w535:i16)
        n328 = Add(x=w534, y=w535) -> (x+y=w533:i16)
        n329 = call <vilib>:"NT Write Number.vi"("Numeric"=w533, "Name"=w532) -> ()  [unwired: 9 in, 1 out]
      }
      event "Test Ring": Value Change {
        # "When a test mode helper value is selected from the ring,\nset the tree item's variable to the string value"
        n330 = event-data() -> ("NewVal"=w542:u16)  [unwired: 1 in]
        n331 = property on="Test Ring" class="Ring (strict)"() -> ("Strings []"=w543:string[])  [unwired: 2 in, 2 out]
        n332 = Index Array(array=w543, index=w542) -> (element=w541:string)
        n333 = call <vilib>:"NT Write String.vi"("String"=w541, "Name"=w540) -> ()  [unwired: 9 in, 1 out]
      }
      event "Rec Mode": Value Change {
        # "Update globals for recording mode and path to read log from.\nClear when logging and let NetworkTables set path for vision to\nuse."
        n334 = event-data() -> ("NewVal"=w552:enum32{"Stop", "Record", "Playback"})  [unwired: 1 in]
        n335 = global write "WPI_DashboardLogging Global.vi" "Logging Filename"(path "") -> ()
        n336 = global write "WPI_DashboardLogging Global.vi" "Recording"(w552) -> ()
        n337 = case shown="\"Playback\"" w552 {
          tunnel: w551 -> [_ w554 w563]
          tunnel: [_ _ w562] -> w549
          tunnel: [_ _ w561] -> _
          tunnel: w547 -> [_ _ w559]
          tunnel: cluster{i32, i32} {-250, 170} -> [_ _ w558]
          tunnel: [_ _ T12 {"Image Size"=TRUE, "Image Type"=TRUE, "Pixel Value"=TRUE, "ROI Information"=TRUE, "Zoom Factor"=FALSE} ("Image Information Shown:All Elements")] -> _
          tunnel: [_ _ TRUE ("Zoom Factor")] -> _
          tunnel: w545 -> [_ _ w555]
          frame Default {
          }
          frame "Stop", "Record" {
            # "Place Window too"
            n338 = invoke class="VI" method="FP.Close"(reference=w554) -> (reference out=w553:refnum<vi>)  [unwired: 2 in, 2 out]
            n339 = invoke class="VI" method="Abort VI"(reference=w553) -> ()  [unwired: 2 in, 3 out]
          }
          frame "Playback" {
            n340 = call "Open Playback Panel.vi"("Offset"=w558, "DB VI Ref"=w559, "Playback in"=w563) -> ("Playback out"=w560:refnum<vi>)  [unwired: 8 in]
            n341 = register-events(w560, w555) -> (reference out=w562:refnum<event-registration>, error out=w561:errorcluster)  [unwired: 2 in]
          }
        }
        n342 = call <vilib>:"WPI_DashboardNT Log FieldName Cache.vi"("Operation"=enum16{"Lookup/Add", "Index", "Clear"}."Clear") -> ()  [unwired: 8 in, 3 out]
      }
      event Panel Close {
        w565 = enum32{"Stop", "Record", "Playback"}."Stop" ("Rec Mode")
        # "Playback window has been closed, abort"
        n343 = event-data() -> ()  [unwired: 1 in, 4 out]
        n344 = local write "Rec Mode"(w565) -> ()
        n345 = global write "WPI_DashboardLogging Global.vi" "Recording"(w565) -> ()
      }
      event Panel Close {
        # "Abort playback window and ourself"
        n346 = event-data() -> ()  [unwired: 1 in, 4 out]
        n347 = invoke class="VI" method="FP.Close"(reference=w569) -> (reference out=w568:refnum<vi>)  [unwired: 2 in, 2 out]
        n348 = invoke class="VI" method="Abort VI"(reference=w568) -> (error out=w567:errorcluster)  [unwired: 2 in, 2 out]
        n349 = invoke class="VI" method="Abort VI"(error in=w567) -> ()  [unwired: 2 in, 3 out]
      }
      event User Event {
        n350 = event-data() -> ("IDs"=w576:cluster{"RPC field ID":u16, "Unique ID":u16}, "String"=w575:string)  [unwired: 1 in]
        n351 = Bundle("IDs"=w576, "String"=w575) -> (w574:T5)  [unwired: 1 in]
        n352 = call <vilib>:"Retrieve RPC Response.vi"("RPC Response"=w574) -> ("Output"=w572:string[][])  [unwired: 10 in]
        n353 = Build Array (concatenate)(w570, w572) -> (w571:string[][])
        n354 = local write "Command Params"(w571) -> ()
        n355 = local write "Cmd Status"("" ("Cmd Status")) -> ()
      }
      event "Tree": Double Click {
        n356 = event-data() -> ("PlatMods"=w582:T15, "Tag"=w579:string)  [unwired: 1 in]
        n357 = Unbundle(w582) -> ("Shift"=w581:bool)  [unwired: 4 out]
        n358 = String Subset(string=w579, length (rest)=1 ("length (rest)")) -> (substring=w578:string)  [unwired: 1 in]
        n359 = Not(x=w581) -> (.not. x?=w580:bool)
        n360 = case shown="\"/\"" w578 {
          tunnel: w579 -> [_ w585]
          tunnel: w580 -> [_ w584]
          frame Default {
          }
          frame "/" {
            n361 = call <vilib>:"NT Update Persistence.vi"("Persistence"=w584, "Name"=w585) -> ()  [unwired: 9 in, 1 out]
          }
        }
      }
    }
  }
  n362 = local write "Dashboard Tab"(T1."Drive" ("Dashboard Tab")) -> ()
  n363 = while {
    stop <- FALSE stop-if-true
    n364 = event shown="[0] \"Left Sidebar Mini\", \"Match Ready\", \"Developer Settings\", \"Boolean 4\": Mouse Enter" {
      selector: _ -> [_ _]
      dyn-events: _ -> [_ _]
      timeout: _ -> [_ _]
      event "Left Sidebar Mini", "Match Ready", "Developer Settings", "Boolean 4": Mouse Enter {
        n365 = event-data() -> ()  [unwired: 1 in, 4 out]
        n366 = property on="Left Sidebar Expanded" class="Bool (strict)"("Visible"=TRUE) -> ()  [unwired: 2 in, 2 out]
        n367 = property on="Match Ready" class="Bool (strict)"("Visible"=TRUE) -> ()  [unwired: 2 in, 2 out]
        n368 = property on="Developer Settings" class="Bool (strict)"("Visible"=TRUE) -> ()  [unwired: 2 in, 2 out]
        n369 = property on="Online Mode" class="Bool (strict)"("Visible"=TRUE) -> ()  [unwired: 2 in, 2 out]
      }
      event "Left Sidebar Expanded": Mouse Leave {
        n370 = event-data() -> ()  [unwired: 1 in, 4 out]
        n371 = property on="Left Sidebar Expanded" class="Bool (strict)"("Visible"=FALSE) -> ()  [unwired: 2 in, 2 out]
        n372 = property on="Match Ready" class="Bool (strict)"("Visible"=FALSE) -> ()  [unwired: 2 in, 2 out]
        n373 = property on="Developer Settings" class="Bool (strict)"("Visible"=FALSE) -> ()  [unwired: 2 in, 2 out]
        n374 = property on="Online Mode" class="Bool (strict)"("Visible"=FALSE) -> ()  [unwired: 2 in, 2 out]
      }
    }
  }
  n375 = property on="On/Off" class="Bool (strict)"("Visible"=w23) -> ()  [unwired: 2 in, 2 out]
  n376 = property on="Motor" class="Clust (strict)"("Visible"=w23) -> ()  [unwired: 2 in, 2 out]
  n377 = property on="Progress" class="Clust (strict)"("Visible"=w23) -> ()  [unwired: 2 in, 2 out]
  n378 = property on="Test Ring" class="Ring (strict)"("Visible"=w23) -> ()  [unwired: 2 in, 2 out]
  n379 = property on="Rev/Fwd" class="Clust (strict)"("Visible"=w23) -> ()  [unwired: 2 in, 2 out]
  n380 = while {
    tunnel: u16 1741 ("timeout ms (25000)") -> [w596]
    stop <- FALSE stop-if-true
    n381 = TCP Create Listener(10:w596) -> (0:w595:errorcluster, 3:w597:refnum<k5>)  [unwired: 4 in, 1 out]
    n382 = case shown="No Error" w595 {
      selector: w595 -> [w599 _]
      tunnel: w597 -> [w600 _]
      frame No Error {
        n383 = while {
          tunnel: w600 -> [w603]
          tunnel: w599 -> [w602]
          stop <- FALSE stop-if-true
          n384 = TCP Wait On Listener(8:w602, 11:w603) -> (0:w604:errorcluster, 4:w605:refnum<k5>)  [unwired: 2 in, 3 out]
          n385 = local write "TCP"(w605) -> ()
          n386 = case shown="No Error" w604 {
            frame No Error {
            }
            frame Error {
              n387 = Wait (ms)(milliseconds to wait=u32 1000) -> ()  [unwired: 1 out]
            }
          }
        }
      }
      frame Error {
        n388 = Wait (ms)(milliseconds to wait=u32 1000) -> ()  [unwired: 1 out]
      }
    }
  }
  n389 = local write "Command Selection"(u16 0 ("milliseconds to wait")) -> ()
  n390 = local write "Command Params"(string[][] [] ("Command Params")) -> ()
  n391 = global write "WPI_DashboardLogging Global.vi" "Recording"(w42) -> ()
  n392 = local write "Rec Mode"(w42) -> ()
  n393 = call <vilib>:"NT Write String.vi"("String"="Select Auto", "Name"="Auto Selector") -> ()  [unwired: 9 in, 1 out]
